vi "Get View Status.vi"(8 "error in (no error)":errorcluster, 10 "View":string, 11 "GUI Container View in":refnum<class "GUI Container.lvclass">) -> (0 "error out":errorcluster, 1 "View Found":bool, 2 "View Status":T1, 3 "GUI Container View out":refnum<class "GUI Container.lvclass">)   [LabVIEW 2023, in "GUI Views.lvlib" / "GUI Container.lvclass"]
uses:
  GUI Container.lvclass
  typedefs/View Status.ctl
  <vilib>/ActorFramework/Message Enqueuer/Message Enqueuer.lvclass
  typedefs/View Details.ctl
  typedefs/FP Status.ctl
  GUI Container.lvclass/GUI Container.ctl
  <vilib>/Utility/error.llb/Error Cluster From Error Code.vi
  <vilib>/ErrorRing/Error Ring.xnode
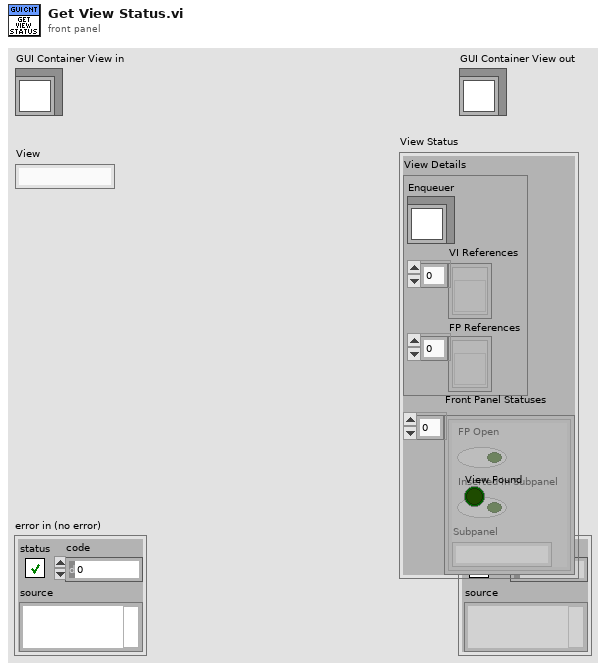
[diagram p1: front panel]
types:
  T1 = typedef "GUI Views.lvlib/GUI Container.lvclass/View Status.ctl" = cluster{"View Details":T2, "Front Panel Statuses":T3[]}
  T2 = typedef "GUI Views.lvlib/GUI Container.lvclass/View Details.ctl" = cluster{"Enqueuer":refnum<class "Message Enqueuer.lvclass">, "VI References":refnum<vi>[], "FP References":refnum<vi>[]}
  T3 = typedef "GUI Views.lvlib/GUI Container.lvclass/FP Status.ctl" = cluster{"FP Open":bool, "Inserted in Subpanel":bool, "Subpanel":string}
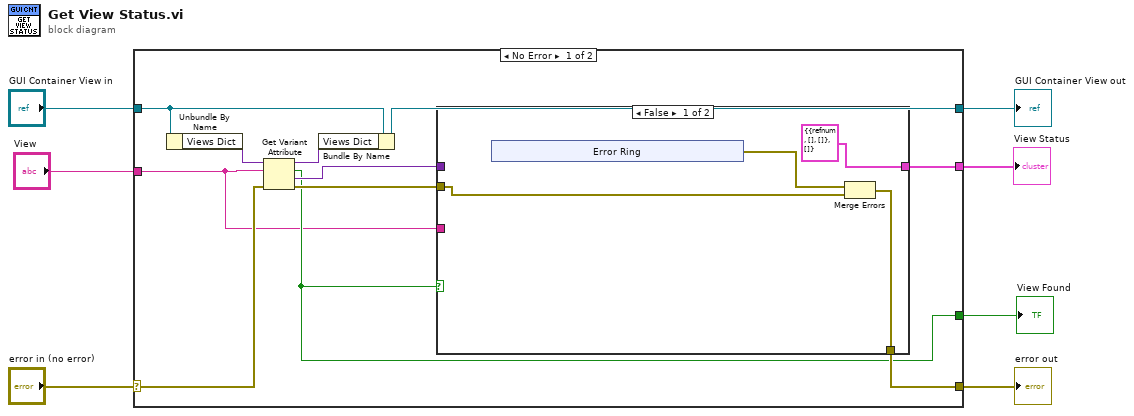
[diagram p0: block diagram]
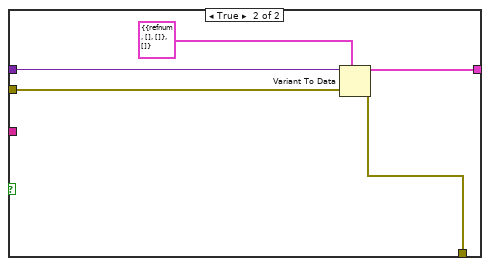
[diagram p2: hidden frame]
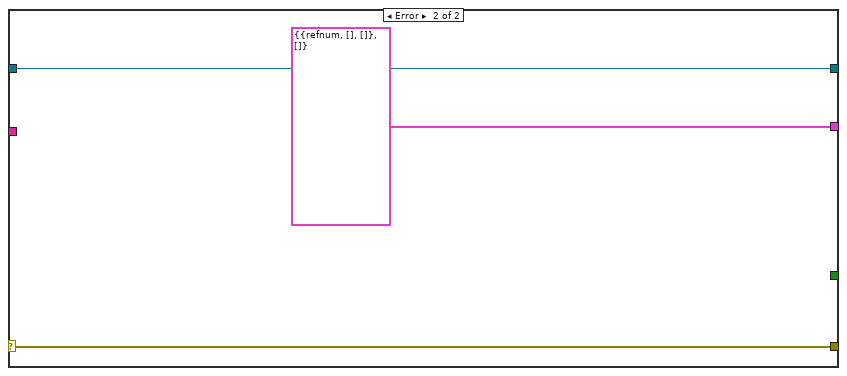
[diagram p3: hidden frame]
diagram:
  n1 = case shown="No Error" "error in (no error)" {
    selector: "error in (no error)" -> [w16 w34]
    tunnel: [w10 w34] -> w6
    tunnel: [w15 w33] -> w4
    tunnel: "GUI Container View in" -> [w18 w33]
    tunnel: "View" -> [w8 _]
    tunnel: [w11 T1 {"View Details"={"Enqueuer"=refnum, "VI References"=[], "FP References"=[]}, "Front Panel Statuses"=[]} ("View State")] -> w2
    tunnel: [w9 _] -> w1
    frame No Error {
      n2 = Unbundle By Name(w18) -> ("Views Dict"=w17:variant)
      n3 = Get Variant Attribute(Variant=w17, name=w8, error in=w16) -> (duplicate Variant=w14:variant, found=w9:bool, value=w12:variant, error out=w13:errorcluster)  [unwired: 1 in]
      n4 = Bundle By Name(cluster=w18, "Views Dict"=w14) -> (w15:refnum<class "GUI Container.lvclass">)
      n5 = case shown="False" w9 {
        tunnel: w13 -> [w19 w31]
        tunnel: w12 -> [_ w30]
        tunnel: [T1 {"View Details"={"Enqueuer"=refnum, "VI References"=[], "FP References"=[]}, "Front Panel Statuses"=[]} ("View State") w28] -> w11
        tunnel: [w22 w27] -> w10
        tunnel: w8 -> [_ _]
        frame False {
          n6 = xnode "Error Ring"() -> ("error out"=w20:errorcluster)
          n7 = Merge Errors(w20, w19) -> (w22:errorcluster)
        }
        frame True {
          n8 = Variant To Data(error in=w31, type=T1 {"View Details"={"Enqueuer"=refnum, "VI References"=[], "FP References"=[]}, "Front Panel Statuses"=[]} ("View State"), Variant=w30) -> (data=w28:T1, error out=w27:errorcluster)
        }
      }
    }
    frame Error {
    }
  }
  "error out" <- w6
  "GUI Container View out" <- w4
  "View Status" <- w2
  "View Found" <- w1
